vi "Gas Flow - TMAl #1.vi"() -> ()   [LabVIEW 2011]
panel:
  out "Meter 7":dbl(knob) scale=0.0..200.0
  out "Meter 5":dbl(knob) scale=0.0..200.0
  out "Meter 4":dbl(knob) scale=0.0..2000.0
  out "Meter 3":dbl(knob) scale=0.0..2000.0
  in  "Tank":dbl(slide) scale=0.0..200.0
  in  "Tank 4":dbl(slide) scale=0.0..2000.0
  in  "Tank 3":dbl(slide) scale=0.0..200.0
  in  "Tank 2":dbl(slide) scale=0.0..2000.0
  in  "42":bool caption="49"
  in  "41":bool caption="49"
  in  "13":bool caption="49"
  in  "14":bool caption="49"
  in  "14":bool caption="49"
  in  "63":bool caption="49"
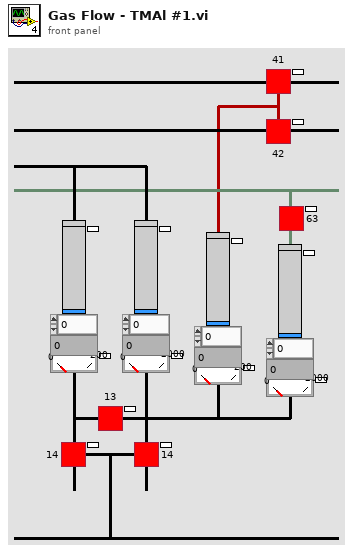
[diagram p1: front panel]
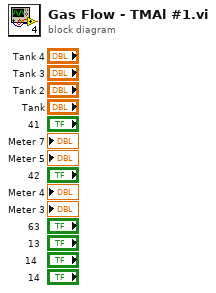
[diagram p0: block diagram]
diagram:
